vi "RichToFlatni_protobuf_types_WaveformAttributeValue.vi"(5 "OutputClusterType":T1, 11 "InputCluster":T2) -> (3 "OutputCluster":T1)   [LabVIEW 2020, in "ni.protobuf.types.lvlib"]
uses:
  ni.protobuf.types.lvlib
  ni_protobuf_types_WaveformAttributeValue.ctl
  ni_protobuf_types_WaveformAttributeValue_attribute/ni_protobuf_types_WaveformAttributeValue_attribute.lvclass
  ni_protobuf_types_WaveformAttributeValue_Flat.ctl
  ni_protobuf_types_WaveformAttributeValue_attribute/ni_protobuf_types_WaveformAttributeValue_attribute.lvclass/ni_protobuf_types_WaveformAttributeValue_attribute.ctl
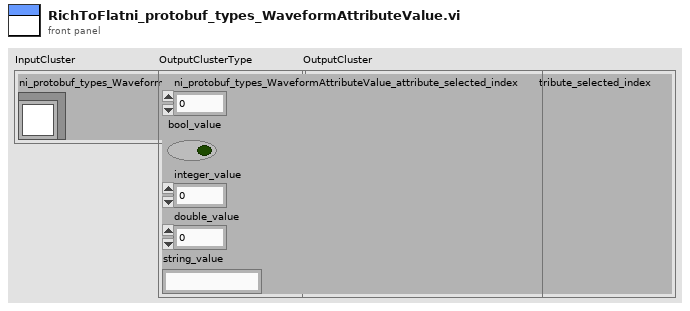
[diagram p1: front panel]
types:
  T1 = typedef "ni.protobuf.types.lvlib/ni_protobuf_types_WaveformAttributeValue_Flat.ctl" = cluster{"ni_protobuf_types_WaveformAttributeValue_attribute_selected_index":i32, "bool_value":bool, "integer_value":i32, "double_value":dbl, "string_value":string}
  T2 = typedef "ni.protobuf.types.lvlib/ni_protobuf_types_WaveformAttributeValue.ctl" = cluster{"ni_protobuf_types_WaveformAttributeValue_attribute":refnum<class "ni_protobuf_types_WaveformAttributeValue_attribute.lvclass">}
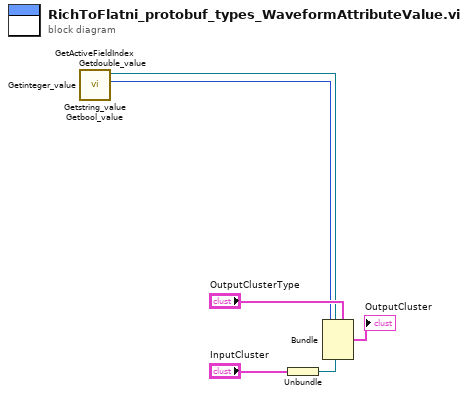
[diagram p0: block diagram]
diagram:
  n1 = Unbundle "Unbundle"("InputCluster") -> ("ni_protobuf_types_WaveformAttributeValue_attribute"=w6:refnum<class "ni_protobuf_types_WaveformAttributeValue_attribute.lvclass">)
  n2 = call "Getstring_value.vi"("OneOfTemplate in"=w6) -> ("Get_Val"=w1:string)  [unwired: 8 in, 2 out]
  n3 = call "Getdouble_value.vi"("OneOfTemplate in"=w6) -> ("Get_Val"=w2:dbl)  [unwired: 8 in, 2 out]
  n4 = call "Getinteger_value.vi"("OneOfTemplate in"=w6) -> ("Get_Val"=w3:i32)  [unwired: 8 in, 2 out]
  n5 = call "Getbool_value.vi"("OneOfTemplate in"=w6) -> ("Get_Val"=w4:bool)  [unwired: 8 in, 2 out]
  n6 = call "GetActiveFieldIndex.vi"("OneOfTemplate in"=w6) -> ("Active Field Index"=w5:i32)  [unwired: 8 in, 2 out]
  n7 = Bundle "Bundle"(cluster="OutputClusterType", "ni_protobuf_types_WaveformAttributeValue_attribute_selected_index"=w5, "bool_value"=w4, "integer_value"=w3, "double_value"=w2, "string_value"=w1) -> (→"OutputCluster":T1)
